vi "Create.vi"(8 "error in (no error)":errorcluster, 10 "JSON":string) -> (0 "error out":errorcluster, 3 "JSON Routing Channel Template out":refnum<class "JSON Routing Channel Template.lvclass">)   [LabVIEW 2020, in "Routing Templates.lvlib" / "JSON Routing Channel Template.lvclass"]
uses:
  JSON Routing Channel Template.lvclass
  JSON Routing Channel Template.lvclass/JSON Routing Channel Template.ctl
  JSON Routing Channel.ctl
  Connection Lookups/2010 Connection Lookup/2010 Connection Lookup.lvclass
  <vilib>/ErrorRing/Error Ring.xnode
  <vilib>/Utility/error.llb/Error Cluster From Error Code.vi
  C:/Users/mjacobso/Desktop/SCM/Routing-Faulting/Source/Routing and Faulting/Routing Templates/Connection Lookups/Abstract Connection Lookup/Abstract Connection Lookup.lvclass
  C:/Users/mjacobso/Desktop/SCM/Routing-Faulting/Source/Routing and Faulting/Routing Templates/Connection Lookups/2010 Connection Lookup/2010 Connection Lookup.lvclass
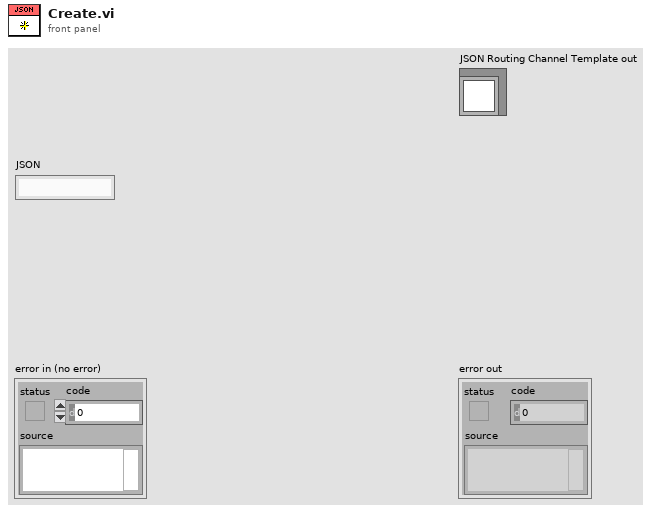
[diagram p1: front panel]
types:
  T1 = typedef "Routing Templates.lvlib/JSON Routing Channel Template.lvclass/JSON Routing Channel.ctl" = cluster{"Routing Channel Name":string, "Module":string, "State Configurations":cluster{"Name":string, "Description":string, "Value":i32, "Connection List":cluster{"Channel":string, "Connection Type":string}[]}[]}
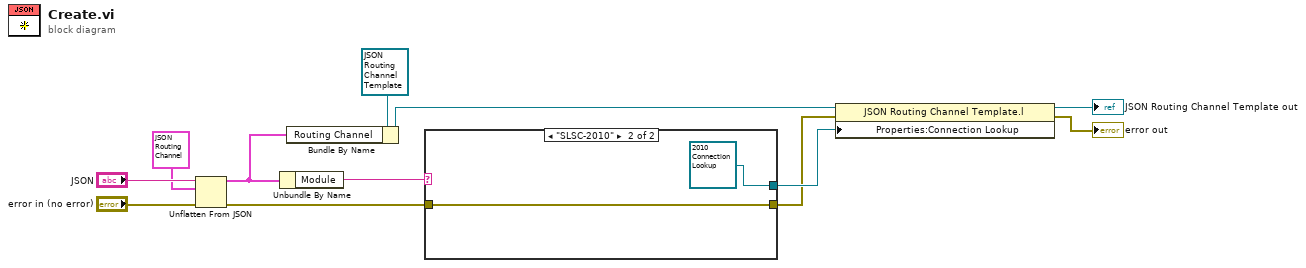
[diagram p0: block diagram]
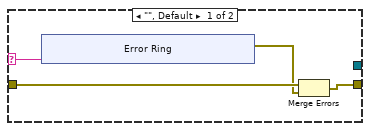
[diagram p2: hidden frame]
diagram:
  n1 = Unflatten From JSON(JSON string="JSON", type and defaults=T1 {"Routing Channel Name"="", "Module"="", "State Configurations"=[{"Name"="", "Description"="", "Value"=-1, "Connection List"=[{"Channel"="", "Connection Type"=""}, {"Channel"="", "Connection Type"=""}]}]} ("Routing Channel"), error in (no error)="error in (no error)") -> (value=w6:T1, error out=w3:errorcluster)  [unwired: 4 in]
  n2 = Unbundle By Name(w6) -> ("Module"=w5:string)
  n3 = Bundle By Name(cluster=refnum<class "JSON Routing Channel Template.lvclass"> refnum ("JSON Routing Channel Template in"), "Routing Channel"=w6) -> (w8:refnum<class "JSON Routing Channel Template.lvclass">)
  n4 = case shown="\"SLSC-2010\"" w5 {
    selector: w5 -> [w16 _]
    tunnel: [_ refnum<class "2010 Connection Lookup.lvclass"> refnum ("Routing Templates.lvlib:2010 Connection Lookup.lvclass")] -> w4
    tunnel: w3 -> [w15 w24]
    tunnel: [w13 w24] -> w2
    frame "", Default {
      n5 = xnode "Error Ring"("parameter 0"=w16) -> ("error out"=w14:errorcluster)
      n6 = Merge Errors(w15, w14) -> (w13:errorcluster)
    }
    frame "SLSC-2010" {
    }
  }
  n7 = property class="JSON Routing Channel Template.l"(reference=w8, error in=w2, "Properties:Connection Lookup"=w4) -> (reference out=→"JSON Routing Channel Template out":refnum<class "JSON Routing Channel Template.lvclass">, error out=→"error out":errorcluster)
